vi "NF WF1973_74 OPER Even.vi"(8 "error in (no error)":errorcluster caption="Error IN", 10 "Channel(Unavailable)":u16(ring) items=["Unavailable", "Ch1", "Ch2"], 11 "VISAsession":refnum<visa-resource-name>) -> (0 "error out":errorcluster caption="Error OUT", 2 "Query Event":i32=999, 3 "CopyVISAsession":refnum<visa-resource-name>)   [LabVIEW 2010]
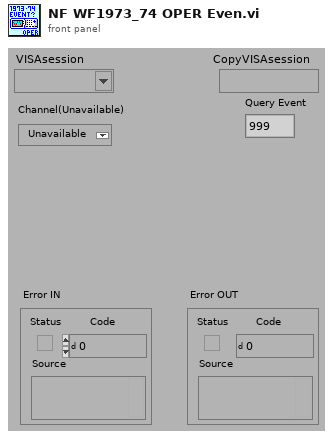
[diagram p1: front panel]
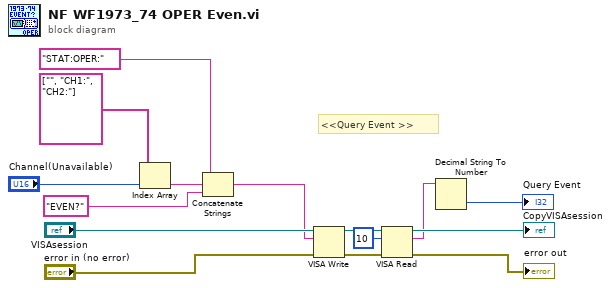
[diagram p0: block diagram]
diagram:
  # "<<Query Event >>"
  n1 = Index Array(array=string[] ["", "CH1:", "CH2:"], index="Channel(Unavailable)") -> (element=w7:string)
  n2 = Concatenate Strings("STAT:OPER:" ("文字列"), w7, "EVEN?" ("文字列")) -> (w1:string)
  n3 = VISA Write(VISA resource name="VISAsession", write buffer=w1, error in (no error)="error in (no error)") -> (VISA resource name out=w4:refnum<visa-resource-name>, error out=w5:errorcluster)  [unwired: 1 out]
  n4 = VISA Read(VISA resource name=w4, byte count=u32 10 ("バイトカウント（0）"), error in (no error)=w5) -> (VISA resource name out=→"CopyVISAsession":refnum<visa-resource-name>, read buffer=w2:string, error out=→"error out":errorcluster)  [unwired: 1 out]
  n5 = Decimal String To Number(string=w2) -> (number=→"Query Event":i32)  [unwired: 2 in, 1 out]
